vi "Packager Output Files Path.vi"(0 "Project Path":path) -> (4 "Package Path":path)   [LabVIEW 2021, in "Path Functions.lvlib"]
uses:
  Path Functions.lvlib
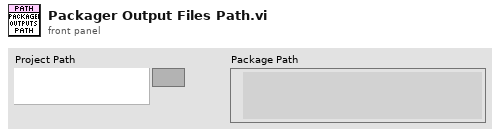
[diagram p1: front panel]
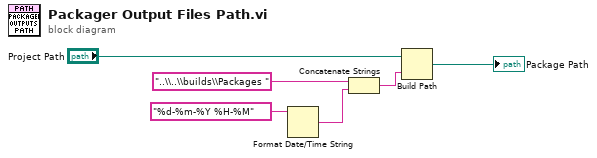
[diagram p0: block diagram]
diagram:
  n1 = Format Date/Time String(time format string (%c)="%d-%m-%Y %H-%M") -> (date/time string=w5:string)  [unwired: 2 in]
  n2 = Concatenate Strings("..\\..\\builds\\Packages ", w5) -> (w1:string)
  n3 = Build Path(base path="Project Path", name or relative path=w1) -> (appended path=→"Package Path":path)
